vi "FMA1600A Main.vi"() -> ()   [LabVIEW 2016]
uses:
  Type Definitions/FMA1600A Data.ctl
  Type Definitions/FMA1600A Gas Type.ctl
  Type Definitions/FMA1600A Commands.ctl
  <vilib>/Utility/file.llb/Write To Spreadsheet File (string).vi
  Yokogawa WT500/Type Definitions/WT500 Wiring Control.ctl
panel:
  in  "stop 2":bool
  out "Data Array":string[][](array[string])
  in  "VISA Input":refnum<visa-resource-name>
  in  "Use Data Save":bool
  in  "Scan Rate (mS)":u32=1000
  in  "file path (dialog if empty)":path=path "C:/Data/FMA1600A.csv"
  in  "Tab Control":enum32{"Page 1", "Page 2"}(tab)
  out "error out":errorcluster
  in  "error in (no error)":errorcluster
  in  "Unit ID":string="A"
  in  "FMA1600A Commands":T1="*@="
  in  "Gas Type":T2="2"
  out "Raw FMA1600A Data":string
  out "FMA1600A Gas Data":T3
  in  "stop":bool
  in  "VISA resource name":refnum<visa-resource-name>="COM3"
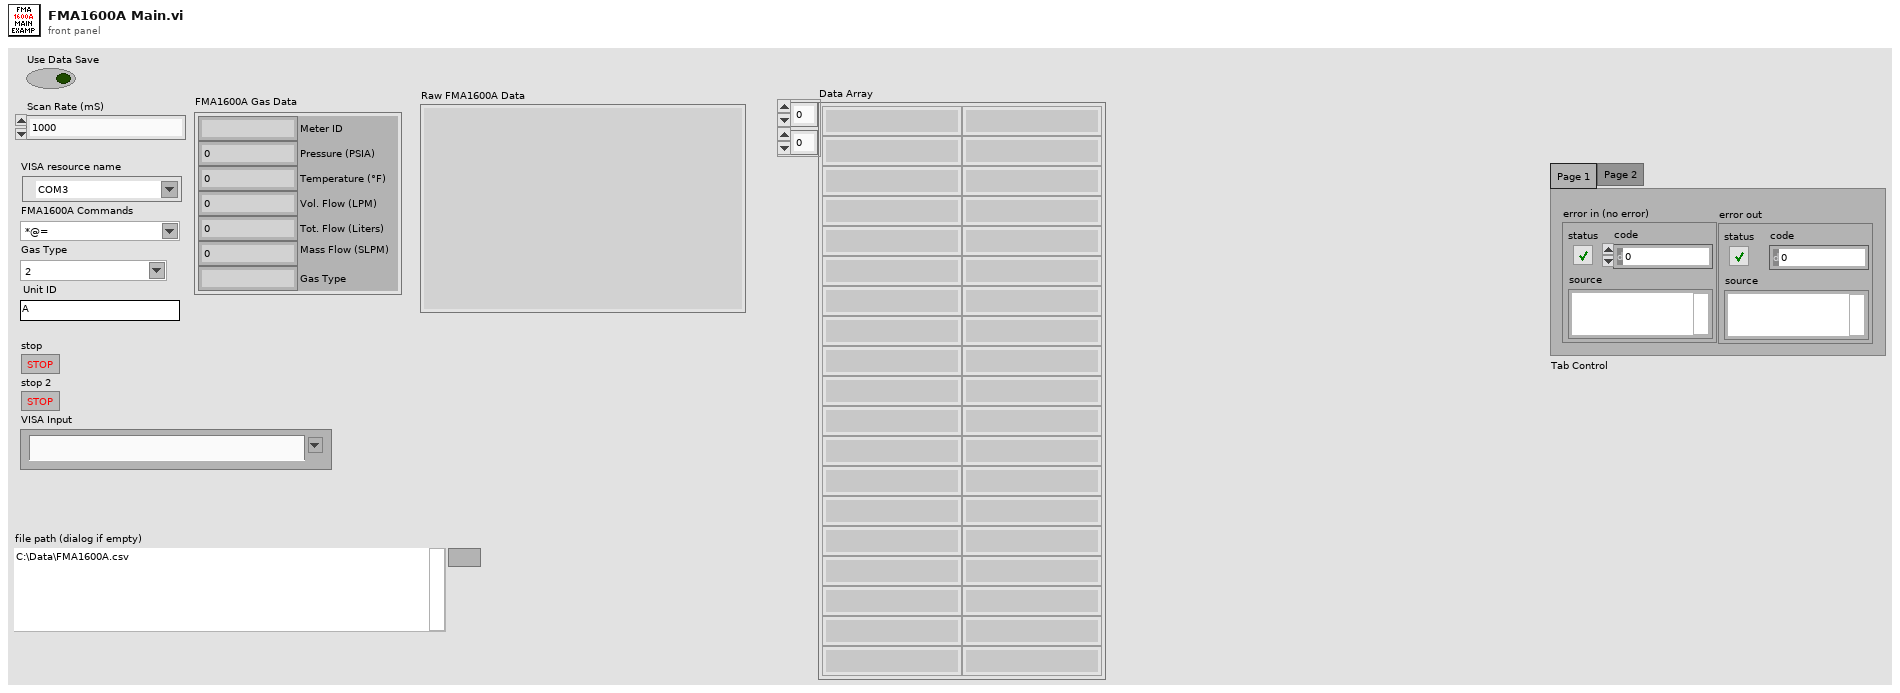
[diagram p1: front panel]
types:
  T1 = typedef "FMA1600A Commands.ctl" = string
  T2 = typedef "FMA1600A Gas Type.ctl" = string
  T3 = typedef "FMA1600A Data.ctl" = cluster{"Pressure (PSIA)":dbl, "Temperature (°F)":dbl, "Vol. Flow (LPM)":dbl, "Mass Flow (SLPM)":dbl, "Gas Type":string, "Tot. Flow (Liters)":dbl, "Meter ID":string}
  T4 = typedef "WT500 Wiring Control.ctl" = u16
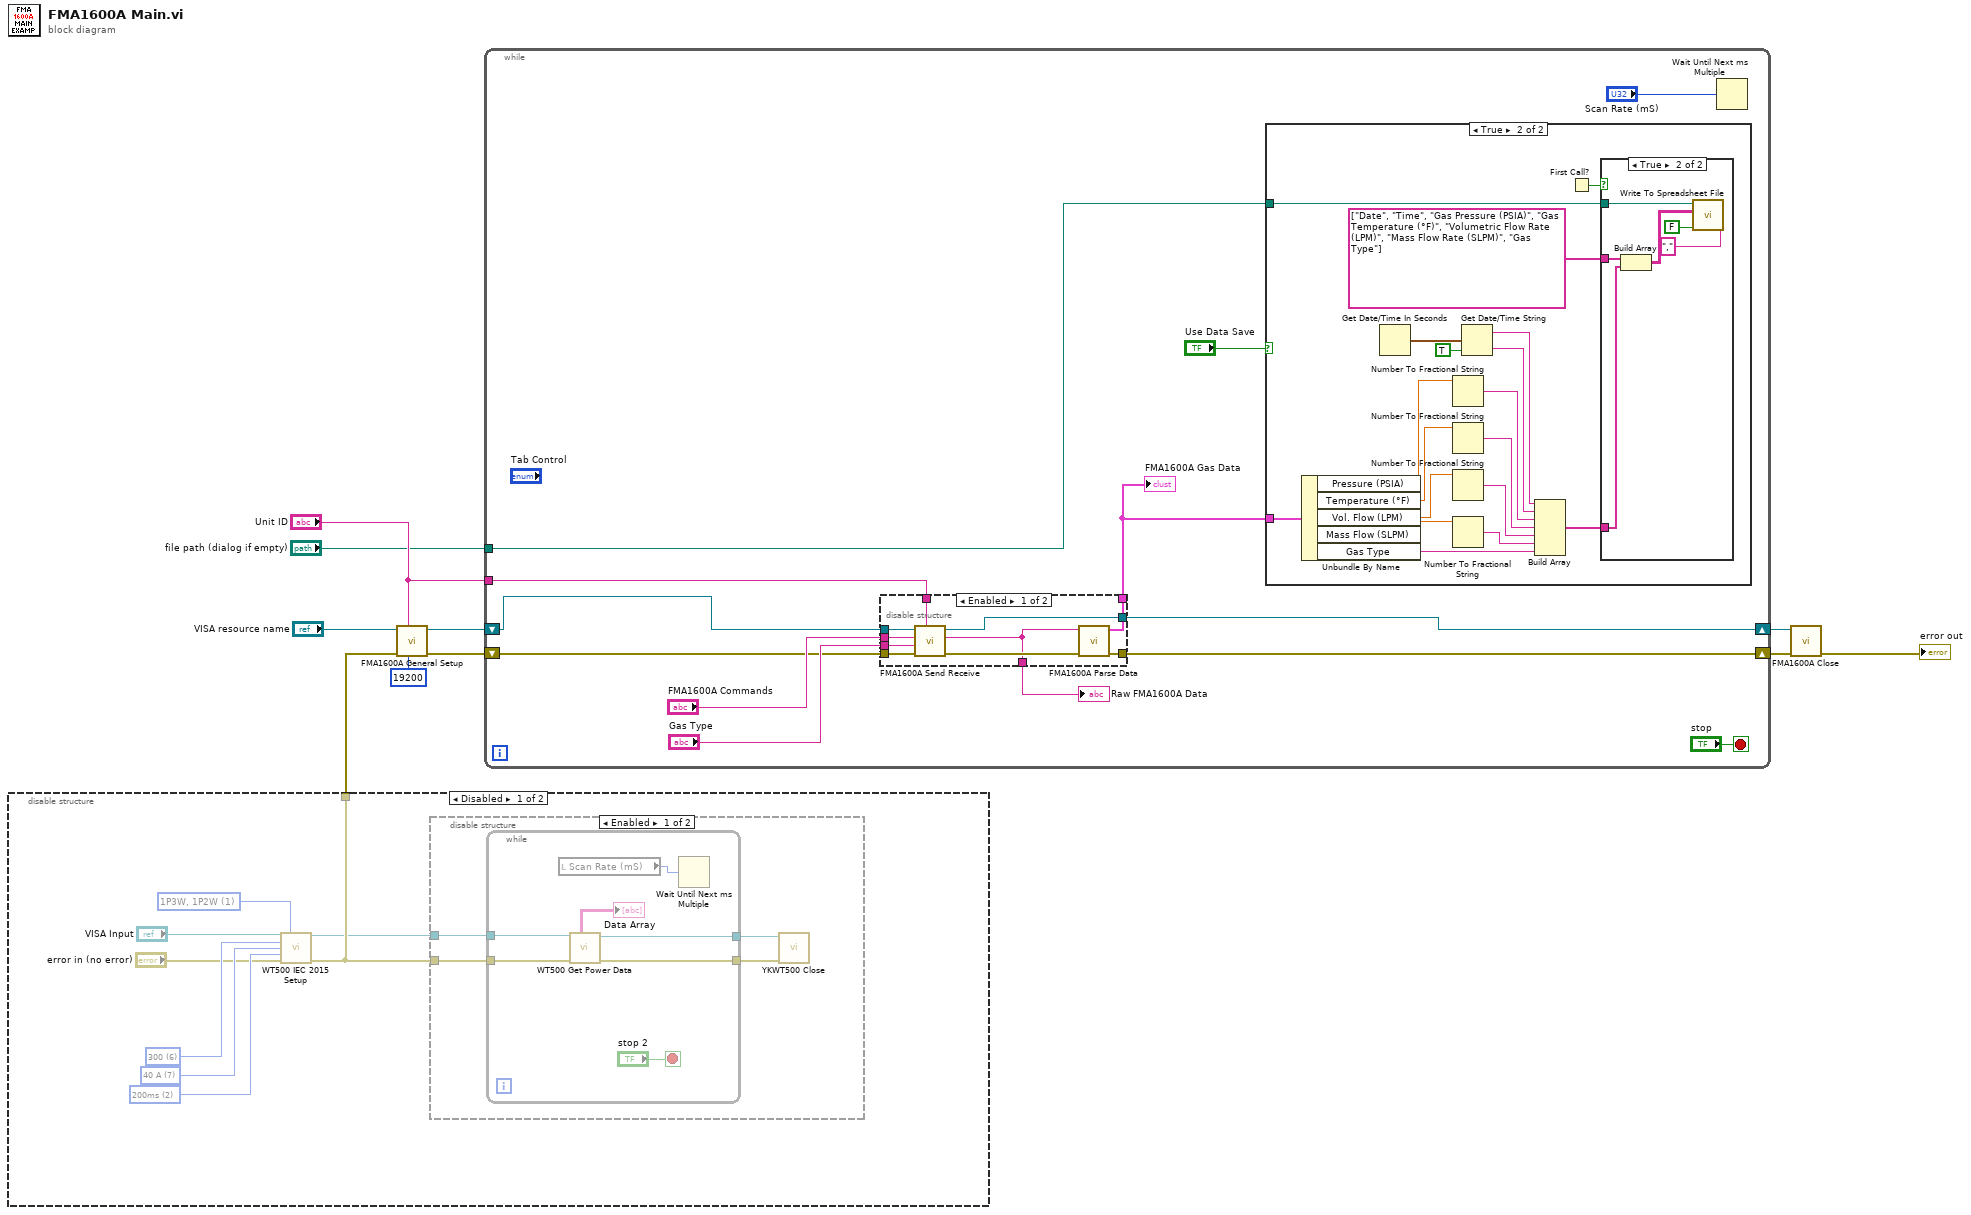
[diagram p0: block diagram]
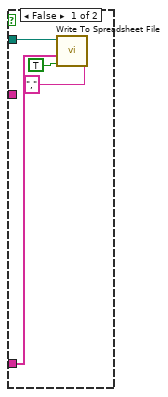
[diagram p6: hidden frame]
diagram:
  n1 = disable-structure shown="Disabled" {
    disable-tunnel: [w13 _] -> w2
    frame Disabled {
      w15 = u16 2 items=["-", "100ms", "200ms", "500ms", "1s", "2s", "5s"] ("Update Rate (3: 500ms)")
      w16 = u16 7 items=["AUTO", "500 mA", "1 A", "2 A", "5 A", "10 A", "20 A", "40 A", "S-AUTO", "50 mV", "100 mV", "200 mV", "500 mV", "1 V", "2 V", "5 V", "10 V", "250 mA", "500 mA", "1 A", "2.5 A", "5 A", "10 A", "20 A", "25 mV", "50 mV", "100 mV", "250 mV", "500 mV", "1 V", "2.5 V", "5 V"] ("I Range (7: 40A)")
      w17 = u16 6 items=["AUTO", "15", "30", "60", "100", "150", "300", "600", "1000", "7.5", "15", "30", "50", "75", "150", "300", "500"] ("V Range (8: 1000V)")
      w18 = T4 1 items=["1P2W, 1P2W, 1P2W", "1P3W, 1P2W", "3P3W, 1P2W", "1P2W, 1P3W", "1P2W, 3P3W", "3P4W", "3V3A"] ("Wiring (0: 1P2W, 1P2W, 1P2W)")
      n2 = call "WT500 IEC 2015 Setup.vi"("VISA Input"="VISA Input", "Wiring (0: 1P2W, 1P2W, 1P2W)"=w18, "V Range (8: 1000V)"=w17, "I Range (7: 40A)"=w16, "Update Rate (3: 500ms)"=w15, "Error In"="error in (no error)") -> ("VISA resource name out"=w11:refnum<visa-resource-name>, "Error Out"=w13:errorcluster)  [unwired: 5 in, 3 out]
      n3 = disable-structure shown="Enabled" {
        disable-tunnel: w11 -> [w22 _]
        disable-tunnel: w13 -> [w19 _]
        frame Enabled {
          n4 = while {
            tunnel: w22 -> [w29]
            tunnel: [w28] -> w21
            tunnel: [w27] -> w20
            tunnel: w19 -> [w26]
            stop <- "stop 2" stop-if-true
            n5 = local read "Scan Rate (mS)"() -> (w25:u32)
            n6 = call "WT500 Get Power Data.vi"("Error In"=w26, "VISA resource name"=w29) -> ("Error Out"=w27:errorcluster, "VISA resource name out"=w28:refnum<visa-resource-name>, "Data Array"=→"Data Array":string[][])  [unwired: 3 in, 3 out]
            n7 = Wait Until Next ms Multiple(millisecond multiple=w25) -> ()  [unwired: 1 out]
          }
          n8 = call "YKWT500 Close.vi"("error in (no error)"=w20, "VISA resource name"=w21) -> ()  [unwired: 9 in, 1 out]
        }
        frame Disabled {
        }
      }
    }
    frame Enabled {
    }
  }
  n9 = call "FMA1600A General Setup.vi"("baud rate (19200)"=u32 19200 ("baud rate (9600)"), "Unit ID"="Unit ID", "error in (no error)"=w2, "VISA Refnum in"="VISA resource name") -> ("error out"=w1:errorcluster, "VISA Refnum out"=w7:refnum<visa-resource-name>)  [unwired: 5 in, 1 out]
  n10 = while {
    shift-right: [w32] -> w8
    shift-left: w7 -> [w42]
    tunnel: "Unit ID" -> [w36]
    tunnel: "file path (dialog if empty)" -> [w34]
    shift-right: [w30] -> w10
    shift-left: w1 -> [w31]
    stop <- "stop" stop-if-true
    n11 = disable-structure shown="Enabled" {
      disable-tunnel: w42 -> [w52 w53]
      disable-tunnel: "FMA1600A Commands" -> [w51 _]
      disable-tunnel: [w49 w54] -> w30
      disable-tunnel: [w48 _] -> w38
      disable-tunnel: "Gas Type" -> [w47 _]
      disable-tunnel: w36 -> [w46 _]
      disable-tunnel: [w45 _] -> w35
      disable-tunnel: [w44 w53] -> w32
      disable-tunnel: w31 -> [w43 w54]
      frame Enabled {
        n12 = call "FMA1600A Send Receive.vi"("Unit ID"=w46, "error in (no error)"=w43, "Gas Type"=w47, "FMA1600A Commands"=w51, "VISA Refnum in"=w52) -> ("error out"=w50:errorcluster, "Raw FMA1600A Data"=w48:string, "VISA Refnum out"=w44:refnum<visa-resource-name>)  [unwired: 4 in]
        n13 = call "FMA1600A Parse Data.vi"("Error In"=w50, "Raw FMA1600A Data"=w48) -> ("Error Out"=w49:errorcluster, "FMA1600A Gas Data"=w45:T3)  [unwired: 7 in]
      }
      frame Disabled {
      }
    }
    "FMA1600A Gas Data" <- w35
    "Raw FMA1600A Data" <- w38
    n14 = case shown="True" "Use Data Save" {
      tunnel: w35 -> [_ w56]
      tunnel: w34 -> [_ w55]
      frame False {
      }
      frame True {
        n15 = Unbundle By Name(w56) -> ("Pressure (PSIA)"=w71:dbl, "Temperature (°F)"=w70:dbl, "Vol. Flow (LPM)"=w69:dbl, "Mass Flow (SLPM)"=w68:dbl, "Gas Type"=w63:string)
        n16 = Get Date/Time In Seconds() -> (seconds since 1Jan1904=w72:timestamp)
        n17 = Number To Fractional String(number=w71) -> (F-format string=w67:string)  [unwired: 3 in]
        n18 = Number To Fractional String(number=w70) -> (F-format string=w66:string)  [unwired: 3 in]
        n19 = Number To Fractional String(number=w69) -> (F-format string=w65:string)  [unwired: 3 in]
        n20 = Number To Fractional String(number=w68) -> (F-format string=w64:string)  [unwired: 3 in]
        n21 = Get Date/Time String(seconds (now)=w72, want seconds? (F)=TRUE) -> (date string=w59:string, time string=w60:string)  [unwired: 1 in]
        n22 = Build Array(w59, w60, w67, w66, w65, w64, w63) -> (w62:string[])
        n23 = First Call?() -> (First Call?: T/F=w57:bool)
        n24 = case shown="True" w57 {
          tunnel: w62 -> [w74 w82]
          tunnel: string[] ["Date", "Time", "Gas Pressure (PSIA)", "Gas Temperature (°F)", "Volumetric Flow Rate (LPM)", "Mass Flow Rate (SLPM)", "Gas Type"] -> [_ w81]
          tunnel: w55 -> [w75 w79]
          frame False {
            n25 = call-poly <vilib>:"Write To Spreadsheet File.vi"("delimiter (\\t)"="," ("delimiter (\\t)"), "append to file? (new file:F)"=TRUE, "1D data"=w74, "file path (dialog if empty)"=w75) -> ()  [unwired: 4 in, 1 out]
          }
          frame True {
            n26 = Build Array(w81, w82) -> (w77:string[][])
            n27 = call-poly <vilib>:"Write To Spreadsheet File.vi"("delimiter (\\t)"="," ("delimiter (\\t)"), "append to file? (new file:F)"=FALSE, "2D data"=w77, "file path (dialog if empty)"=w79) -> ()  [unwired: 4 in, 1 out]
          }
        }
      }
    }
    n28 = Wait Until Next ms Multiple(millisecond multiple="Scan Rate (mS)") -> ()  [unwired: 1 out]
  }
  n29 = call "FMA1600A Close.vi"("error in (no error)"=w10, "VISA Refnum in"=w8) -> ("error out"=→"error out":errorcluster)  [unwired: 9 in]
